vi "email_getTypeMsg.vi"(8 "entrée d'erreur (pas d'erreur)":errorcluster, 11 "trimmed string":string) -> (0 "sortie d'erreur":errorcluster, 2 "content":string, 3 "typeMsg":string)   [LabVIEW 2020]
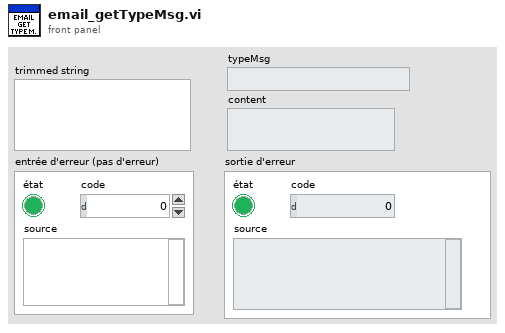
[diagram p1: front panel]
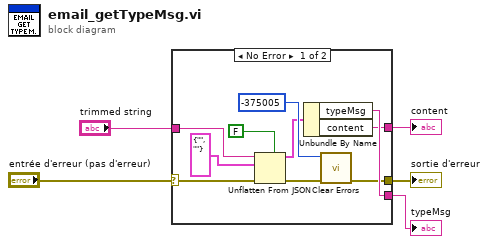
[diagram p0: block diagram]
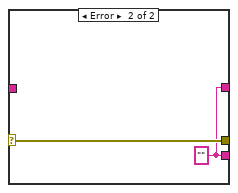
[diagram p2: hidden frame]
diagram:
  n1 = case shown="No Error" "entrée d'erreur (pas d'erreur)" {
    selector: "entrée d'erreur (pas d'erreur)" -> [w15 w17]
    tunnel: [w7 w17] -> w2
    tunnel: [w11 w16] -> w3
    tunnel: "trimmed string" -> [w9 _]
    tunnel: [w6 w16] -> w1
    frame No Error {
      n2 = Unflatten From JSON(enable LabVIEW extensions? (T)=FALSE ("activer les extensions LabVIEW ? (V)"), JSON string=w9, type and defaults=cluster{"typeMsg":string, "content":string} {"typeMsg"="", "content"=""} ("Cluster"), error in (no error)=w15) -> (value=w10:cluster{"typeMsg":string, "content":string}, error out=w13:errorcluster)  [unwired: 3 in]
      n3 = Unbundle By Name(w10) -> ("typeMsg"=w11:string, "content"=w6:string)
      n4 = call <vilib>:"Clear Errors.vi"("error in (no error)"=w13, "specific error code to clear (0: all)"=-375005) -> ("error out"=w7:errorcluster)  [unwired: 4 in, 1 out]
    }
    frame Error {
      w16 = "" ("typeMsg")
    }
  }
  "sortie d'erreur" <- w2
  "typeMsg" <- w3
  "content" <- w1
